vi "Read CN PNG.vi"(8 "error in (no error)":errorcluster, 11 "floder Path":path) -> (0 "error out":errorcluster, 2 "Images":T1[](array[typedef]), 3 "filenames":string[](array[string]))   [LabVIEW 2014]
uses:
  <vilib>/picture/picture.llb/imagedata.ctl
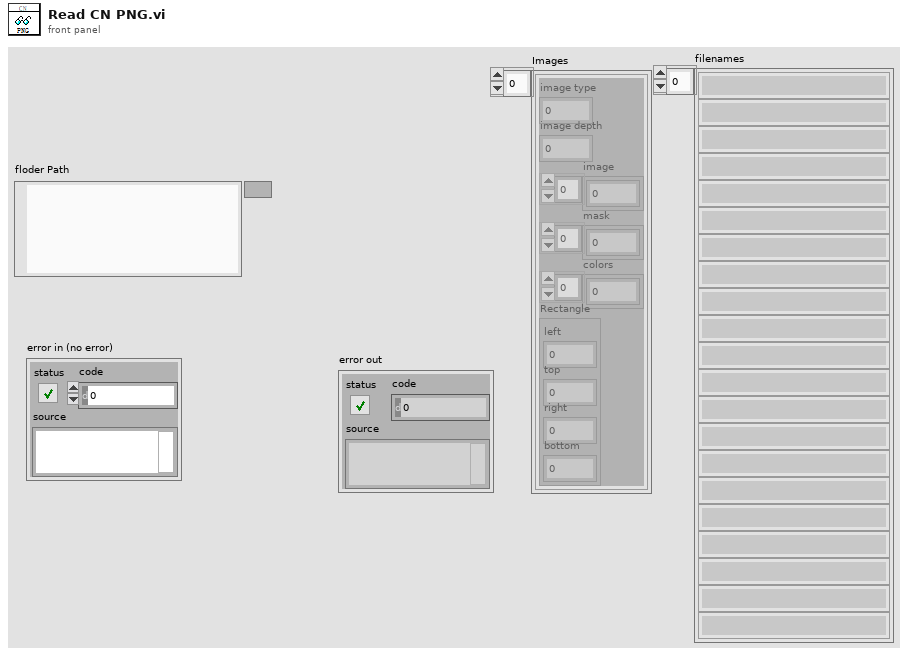
[diagram p1: front panel]
types:
  T1 = typedef "imagedata.ctl" = cluster{"image type":i32, "image depth":i32, "image":u8[], "mask":u8[], "colors":u32[], "Rectangle":cluster{"left":i16, "top":i16, "right":i16, "bottom":i16}}
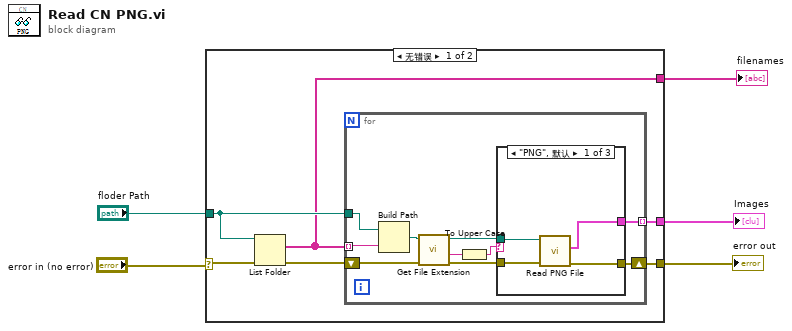
[diagram p0: block diagram]
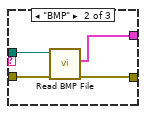
[diagram p2: hidden frame]
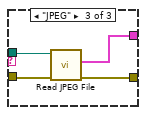
[diagram p3: hidden frame]
diagram:
  n1 = case shown="无错误" "error in (no error)" {
    selector: "error in (no error)" -> [w11 w34]
    tunnel: "floder Path" -> [w9 _]
    tunnel: [w8 _] -> w2
    tunnel: [w7 w34] -> w3
    tunnel: [w6 _] -> w1
    frame No Error {
      n2 = List Folder(path=w9, error in=w11) -> (filenames=w6:string[], error out=w10:errorcluster)  [unwired: 2 in, 2 out]
      n3 = for {
        tunnel: w6 -> [w20] mode=indexing
        tunnel: w9 -> [w21]
        tunnel: [w12] -> w8 mode=indexing
        shift-right: [w13] -> w7
        shift-left: w10 -> [w18]
        n4 = Build Path(base path=w21, name or relative path=w20) -> (appended path=w19:path)
        n5 = call <vilib>:"Get File Extension.vi"("error in (no error)"=w18, "file"=w19) -> ("error out"=w17:errorcluster, "filename without extension"=w15:string, "dup file"=w16:path)  [unwired: 6 in, 1 out]
        n6 = To Upper Case(1:w15) -> (0:w14:string)
        n7 = case shown="\"PNG\", 默认" w14 {
          tunnel: w17 -> [w25 w29 w33]
          tunnel: w16 -> [w24 w28 w32]
          tunnel: [w23 w27 w31] -> w13
          tunnel: [w22 w26 w30] -> w12
          frame "PNG", Default {
            n8 = call <vilib>:"Read PNG File.vi"("error in (no error)"=w25, "path to PNG file"=w24) -> ("error out"=w23:errorcluster, "image data"=w22:T1)  [unwired: 7 in, 1 out]
          }
          frame "BMP" {
            n9 = call <vilib>:"Read BMP File.vi"("error in (no error)"=w29, "path to BMP file"=w28) -> ("error out"=w27:errorcluster, "image data"=w26:T1)  [unwired: 7 in, 1 out]
          }
          frame "JPEG" {
            n10 = call <vilib>:"Read JPEG File.vi"("error in (no error)"=w33, "path to JPEG file"=w32) -> ("error out"=w31:errorcluster, "image data"=w30:T1)  [unwired: 7 in, 1 out]
          }
        }
      }
    }
    frame Error {
    }
  }
  "error out" <- w3
  "Images" <- w2
  "filenames" <- w1
